vi "Write Simple Sequencer Configuration.vi"(8 "error in (no error)":errorcluster, 10 "Configuration":T1, 11 "Simple Sequencer in":refnum<class "Simple Sequencer.lvclass">) -> (0 "error out":errorcluster, 3 "Simple Sequencer out":refnum<class "Simple Sequencer.lvclass">)   [LabVIEW 2018, in "Simple Sequencer.lvclass"]
uses:
  Simple Sequencer.lvclass
  C:/github/2018/LabActor/Template Module/Template Module.lvclass
  Simple Sequencer Configuration.ctl
  Template Module/Template Module.lvclass/Template Module.ctl
  Template Module/Write Configuration.vi
panel:
  # "Primary sequence"
  # "Secondary sequence"
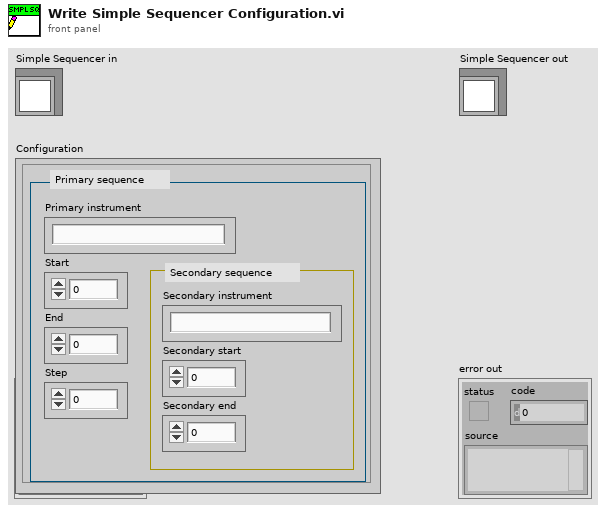
[diagram p1: front panel]
types:
  T1 = typedef "Simple Sequencer Configuration.ctl" = cluster{"Primary instrument":string, "Secondary instrument":string, "Start":dbl, "End":dbl, "Step":dbl, "Secondary start":dbl, "Secondary end":dbl}
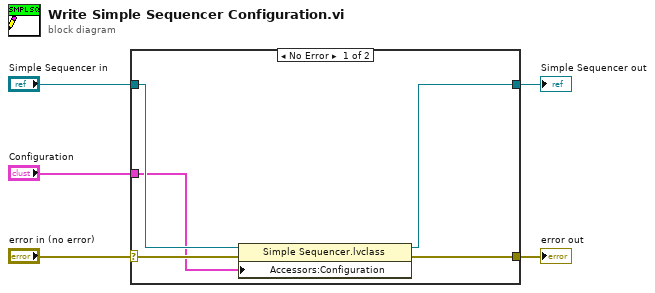
[diagram p0: block diagram]
diagram:
  n1 = case shown="No Error" "error in (no error)" {
    selector: "error in (no error)" -> [w10 w11]
    tunnel: [w9 w11] -> w4
    tunnel: [w7 w12] -> w2
    tunnel: "Simple Sequencer in" -> [w8 w12]
    tunnel: "Configuration" -> [w6 _]
    frame No Error {
      n2 = property class="Simple Sequencer.lvclass"(reference=w8, error in=w10, "Accessors:Configuration"=w6) -> (reference out=w7:refnum<class "Simple Sequencer.lvclass">, error out=w9:errorcluster)
    }
    frame Error {
    }
  }
  "error out" <- w4
  "Simple Sequencer out" <- w2
